vi "Core.vi"(6 "Show FP?":bool, 8 "error in (no error)":errorcluster, 11 "launcher in":refnum<class "launcher.lvclass">) -> (0 "error out":errorcluster, 3 "launcher out":refnum<class "launcher.lvclass">)   [LabVIEW 2021, in "launcher.lvclass"]
uses:
  launcher.lvclass
  <userlib>/S2 Labs/Module Framework/Modules/Base/Module.lvclass
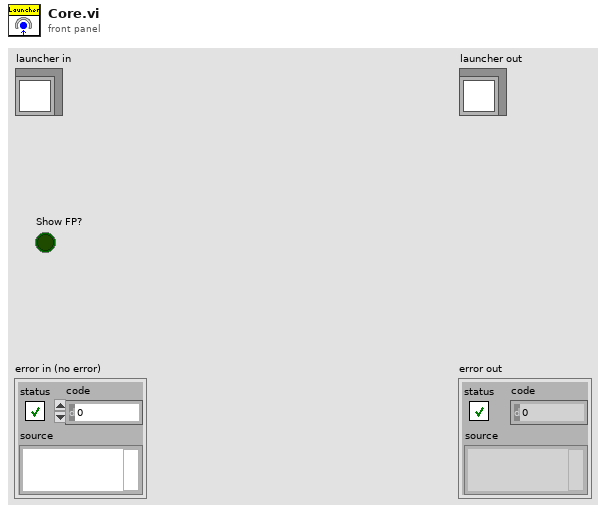
[diagram p1: front panel]
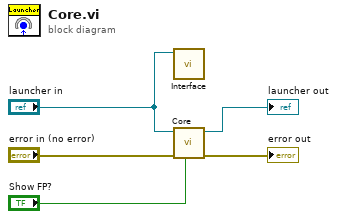
[diagram p0: block diagram]
diagram:
  n1 = call "Interface.vi"("launcher in"="launcher in") -> ()  [unwired: 10 in, 1 out]
  n2 = call-parent "Core.vi"("Show FP?"="Show FP?", "error in (no error)"="error in (no error)", "Module in"="launcher in") -> ("error out"=→"error out":errorcluster, "Module out"=→"launcher out":refnum<class "launcher.lvclass">)  [unwired: 7 in]
